vi "start_by_reference_y.vi"(8 "error in (no error)":errorcluster, 11 "SignalWriterMH110203USBStepperMotor in":refnum<class "SignalWriterMH110203USBStepperMotor.lvclass">) -> (0 "error out":errorcluster, 3 "SignalWriterMH110203USBStepperMotor out":refnum<class "SignalWriterMH110203USBStepperMotor.lvclass">)   [LabVIEW 2010, in "SignalWriterMH110203USBStepperMotor.lvclass"]
uses:
  SignalWriterMH110203USBStepperMotor.lvclass
  <vilib>/Platform/TimedLoop/XDataNode/XDataNode.xnode
  <vilib>/Platform/TimedLoop/XDataNode/timing_clust.ctl
  <vilib>/Platform/TimedLoop/XDataNode/nitl_modes.ctl
  <vilib>/Platform/TimedLoop/XDataNode/wakeup.ctl
  SignalWriterMH110203USBStepperMotor.lvclass/SignalWriterMH110203USBStepperMotor.ctl
  class_data.vi
  common/classes/ErrorController/ErrorController/class_data.vi
  <vilib>/Platform/TimedLoop/XDataNode/XDNodeRunTimeDep.lvlib
  common/classes/ErrorController/ErrorController/ErrorController.lvclass
panel:
  in  "stop_by_reference":bool
  in  "continuous_samples":i32
  in  "start_scanning":bool
  in  "new_position":dbl[](array[numeric])
  in  "pixel_dwell_time":i64
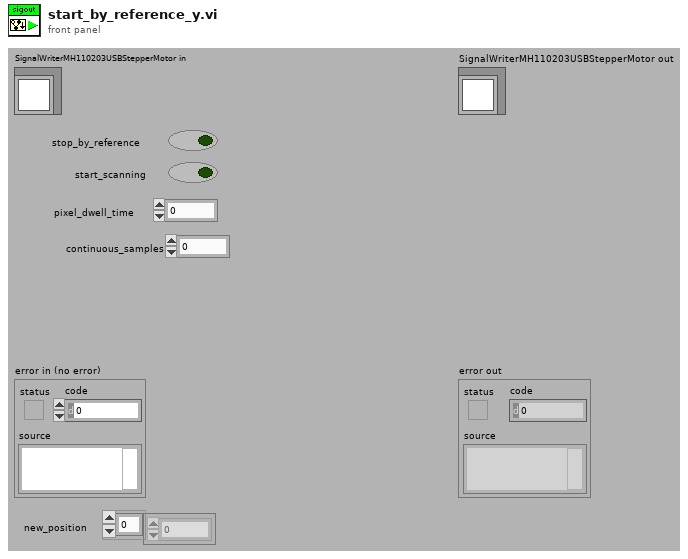
[diagram p1: front panel]
types:
  T1 = typedef "XDNodeRunTimeDep.lvlib/timing_clust.ctl" = cluster{"Expected End [f-1]":u64, "Actual End [f-1]":u64, "Finished Late? [f-1]":bool, "Expected End [i-1]":u64, "Actual End [i-1]":u64, "Finished Late? [i-1]":bool, "Expected Start [i]":u64, "Actual Start [i]":u64, "Expected Start [f]":u64, "Actual Start [f]":u64, "Source Name":string, "Structure Name":string, "Period":i64, "Deadline":i64, "Offset":i64, "Start":i64, "Priority":i32, "Timeout":i32, "Mode":T2, "Wakeup Reason":T3, "Error":errorcluster, "Source Type":string, "Secondary Source Type":string, "Global End Time":u64, "Global Start Time":u64, "Frame Duration":u64, "Iteration Duration":u64, "Assigned CPU":i32, "I/O Scan Engine Mode":u32}
  T2 = typedef "XDNodeRunTimeDep.lvlib/nitl_modes.ctl" = enum32{"No Change", "Process missed periods, maintain original phase", "Discard missed periods, maintain original phase", "Process missed periods, ignore original phase", "Discard missed periods, ignore original phase"}
  T3 = typedef "XDNodeRunTimeDep.lvlib/wakeup.ctl" = enum32{"Normal", "Aborted", "Asynchronous wakeup", "Timing source error", "Timed loop error", "Timeout"}
  T4 = typedef "SignalWriterMH110203USBStepperMotor.lvclass/GoTo Control (uSMC).ctl" = cluster{"Step motor ID":string, "SMname":string, "Backlash":u16, "wait for input sygnal to start":bool, "use slow start/stop":bool, "units name":string, "Maximum speed":dbl, "speed":dbl, "step":u8, "point 1 ticks":i32, "point 2 ticks":i32, "point 1 units":dbl, "point 2 units":dbl, "Limit Switch standoff":dbl, "Zero Value":dbl, "Destination Position":dbl, "force backlash":bool, "power off when stop":bool, "POff delay":dbl, "positioner name":string, "R, Ohm":dbl, "I, mA":dbl, "Positioner's Type":u16, "Reset Direction":bool, "Manufacturer":string, "Model":string, "Scheme":string, "FirmwareVer":string}
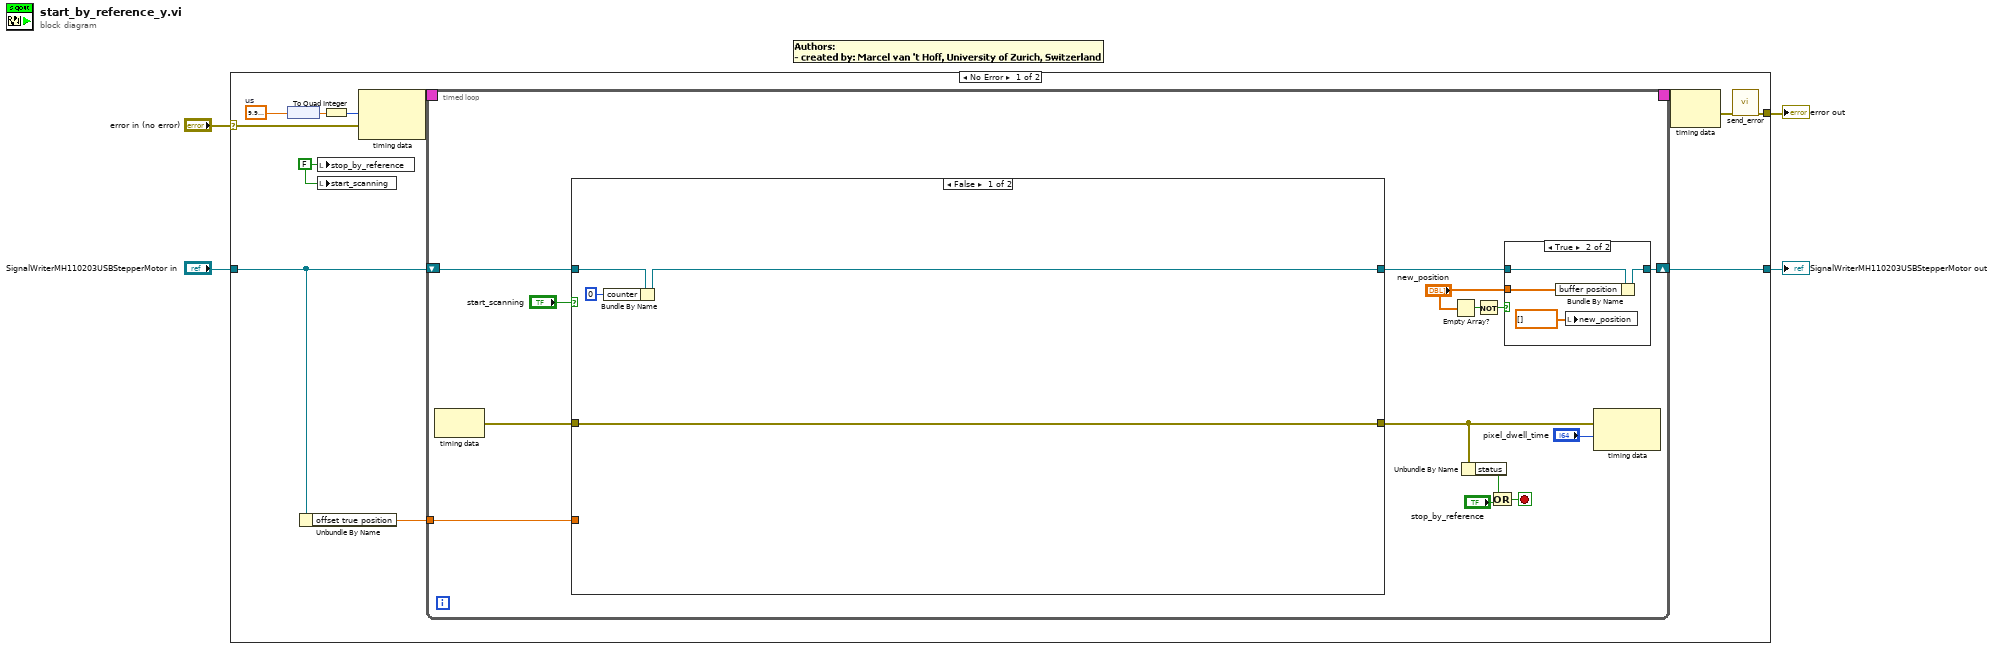
[diagram p0: block diagram]
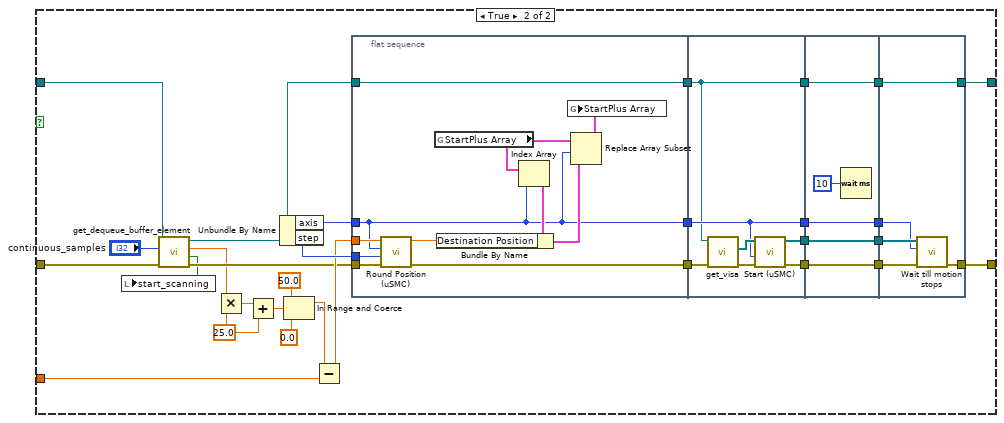
[diagram p3: hidden frame]
diagram:
  n1 = case shown="No Error" "error in (no error)" {
    selector: "error in (no error)" -> [w9 w110]
    tunnel: [w11 w111] -> w2
    tunnel: "SignalWriterMH110203USBStepperMotor in" -> [w6 w111]
    tunnel: [w7 w110] -> w1
    frame No Error {
      w5 = FALSE ("stop_by_reference")
      w10 = dbl[unit] 9.999999999999999e-05  # us
      n2 = node(w10) -> (w16:dbl)
      n3 = Unbundle By Name(w6) -> ("offset true position"=w12:dbl)
      n4 = local write "stop_by_reference"(w5) -> ()
      n5 = local write "start_scanning"(w5) -> ()
      n6 = To Quad Integer(1:w16) -> (0:w13:i64)
      n7 = node-c288(w13, w9) -> (w15:T1)
      n8 = timed-loop {
        timing: w15 -> [_]
        timing-out: [_] -> w14
        tunnel: w12 -> [w30]
        shift-right: [w19] -> w11
        shift-left: w6 -> [w25]
        stop <- w27 stop-if-true
        n9 = node-c288() -> (w26:errorcluster)  [unwired: 1 in]
        n10 = case shown="False" "start_scanning" {
          tunnel: w30 -> [_ w69]
          tunnel: [w36 w68] -> w21
          tunnel: [w39 w67] -> w18
          tunnel: w26 -> [w39 w66]
          tunnel: w25 -> [w37 w65]
          frame False {
            n11 = Bundle By Name(cluster=w37, "counter"=0) -> (w36:refnum<class "SignalWriterMH110203USBStepperMotor.lvclass">)
          }
          frame True {
            w51 = 25.0 ("y")
            n12 = call-dynamic "get_dequeue_buffer_element.vi"("error in (no error)"=w66, "continuous samples?"="continuous_samples", "SignalWriterMH110203USBStepperMotor in"=w65) -> ("error out"=w44:errorcluster, "finished?"=w41:bool, "dequeued element"=w42:dbl, "SignalWriterMH110203USBStepperMotor out"=w43:refnum<class "SignalWriterMH110203USBStepperMotor.lvclass">)  [unwired: 5 in]
            n13 = local write "start_scanning"(w41) -> ()
            n14 = Multiply(x=w42, y=w51) -> (x*y=w49:dbl)
            n15 = Add(x=w49, y=w51) -> (x+y=w50:dbl)
            n16 = Unbundle By Name(w43) -> ("axis"=w47:i32, "step"=w46:u8)
            n17 = In Range and Coerce(upper limit=50.0, x=w50, lower limit=0.0) -> (coerced(x)=w48:dbl)  [unwired: 1 out]
            n18 = Subtract(x=w48, y=w69) -> (x-y=w45:dbl)
            n19 = flat-sequence {
              tunnel: w44 -> [w80]
              tunnel: w45 -> [w79]
              tunnel: w47 -> [w70]
              tunnel: w46 -> [w74]
              tunnel: [w72] -> w64
              tunnel: w43 -> [w72]
              tunnel: [w71] -> w63
              tunnel: [w70] -> w62
              tunnel: w64 -> [w81]
              tunnel: w63 -> [w85]
              tunnel: w62 -> [w82]
              tunnel: [w84] -> w61
              tunnel: [w83] -> w60
              tunnel: [w82] -> w59
              tunnel: [w81] -> w58
              tunnel: w61 -> [w92]
              tunnel: [w92] -> w57
              tunnel: [w91] -> w56
              tunnel: w60 -> [w91]
              tunnel: w59 -> [w89]
              tunnel: [w89] -> w55
              tunnel: [w88] -> w54
              tunnel: w58 -> [w88]
              tunnel: w57 -> [w97]
              tunnel: w56 -> [w96]
              tunnel: w55 -> [w95]
              tunnel: [w94] -> w67
              tunnel: [w93] -> w68
              tunnel: w54 -> [w93]
              frame #0 {
                n20 = call "Round Position (uSMC).vi"("error in"=w80, "Step"=w74, "index"=w70, "Position(value)"=w79) -> ("error out"=w71:errorcluster, "Position(rounded)"=w75:dbl)  [unwired: 6 in]
                n21 = global read "class_data.vi" "StartPlus Array"() -> (w77:T4[])
                n22 = Index Array(array=w77, index=w70) -> (element=w76:T4)
                n23 = Bundle By Name(cluster=w76, "Destination Position"=w75) -> (w78:T4)
                n24 = Replace Array Subset(array=w77, new element=w78, index=w70) -> (w73:T4[])
                n25 = global write "class_data.vi" "StartPlus Array"(w73) -> ()
              }
              frame #1 {
                n26 = call-dynamic "get_visa.vi"("error in (no error)"=w85, "SignalWriterMH110203USBStepperMotor in"=w81) -> ("error out"=w86:errorcluster, "visa array"=w87:refnum<visa-resource-name>[])  [unwired: 6 in, 2 out]
                n27 = call "Start (uSMC).vi"("error in"=w86, "Index"=w82, "Visa Array In"=w87) -> ("error out"=w83:errorcluster, "Visa Array Out"=w84:refnum<visa-resource-name>[])  [unwired: 7 in]
              }
              frame #2 {
                n28 = Wait (ms)(milliseconds to wait=u32 10) -> ()  [unwired: 1 out]
              }
              frame #3 {
                n29 = call "Wait till motion stops.vi"("error in"=w96, "Index"=w95, "Visa Array Out"=w97) -> ("error out"=w94:errorcluster)  [unwired: 5 in, 3 out]
              }
            }
          }
        }
        n30 = Empty Array?(array="new_position") -> (empty?=w23:bool)
        n31 = Unbundle By Name(w18) -> ("status"=w29:bool)
        n32 = Not(x=w23) -> (.not. x?=w22:bool)
        n33 = Or(x=w29, y="stop_by_reference") -> (x .or. y?=w27:bool)
        n34 = case shown="True" w22 {
          tunnel: w21 -> [w31 w35]
          tunnel: [w31 w34] -> w19
          tunnel: "new_position" -> [_ w33]
          frame False {
          }
          frame True {
            n35 = Bundle By Name(cluster=w35, "buffer position"=w33) -> (w34:refnum<class "SignalWriterMH110203USBStepperMotor.lvclass">)
            n36 = local write "new_position"(dbl[] [] ("new_position")) -> ()
          }
        }
        n37 = node-c288(w18, "pixel_dwell_time") -> ()  [unwired: 1 out]
      }
      n38 = node-c288(w14) -> (w8:errorcluster)
      n39 = call "send_error.vi"("error in (no error)"=w8) -> ("error out"=w7:errorcluster)  [unwired: 10 in]
    }
    frame Error {
    }
  }
  "error out" <- w1
  "SignalWriterMH110203USBStepperMotor out" <- w2
